vi "Enable Out CHs.vi"(8 "Error In":errorcluster, 9 "Output CH CTL":T1, 10 "OK Button":bool, 11 "UI Refs in":T2) -> (0 "Error Out":errorcluster, 5 "UI Refs out":T2)   [LabVIEW 2017, in "Waveform-Processing-Custom-Device System Explorer.lvlib"]
uses:
  Waveform-Processing-Custom-Device System Explorer.lvlib
  Types/UI Refs Ctl.ctl
  Shared/Types/OutCHEnum.ctl
  Shared/Waveform-Processing-Custom-Device Shared.lvlib
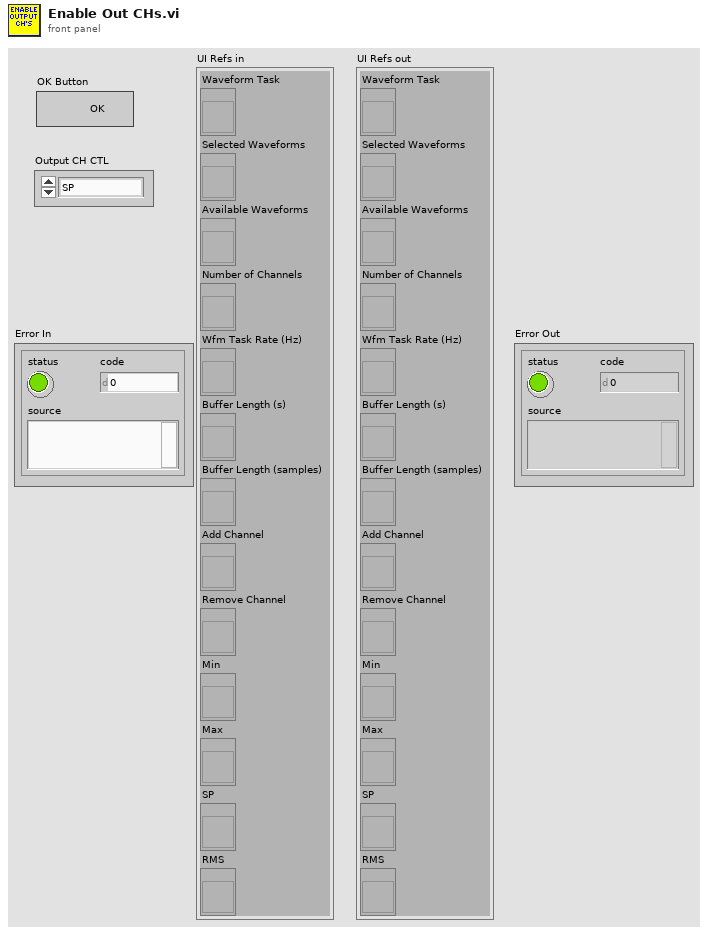
[diagram p1: front panel]
types:
  T1 = typedef "Waveform-Processing-Custom-Device Shared.lvlib/OutCHEnum.ctl" = enum16{"SP", "MIN", "MAX", "RMS"}
  T2 = typedef "Waveform-Processing-Custom-Device Shared.lvlib/UI Refs Ctl.ctl" = cluster{"Waveform Task":refnum<vi>, "Selected Waveforms":refnum<vi>, "Available Waveforms":refnum<vi>, "Number of Channels":refnum<vi>, "Wfm Task Rate (Hz)":refnum<vi>, "Buffer Length (s)":refnum<vi>, "Buffer Length (samples)":refnum<vi>, "Add Channel":refnum<vi>, "Remove Channel":refnum<vi>, "Min":refnum<vi>, "Max":refnum<vi>, "SP":refnum<vi>, "RMS":refnum<vi>}
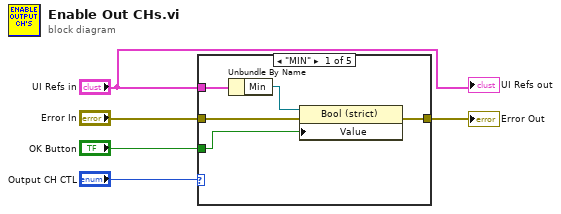
[diagram p0: block diagram]
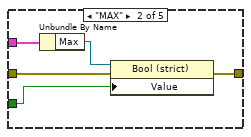
[diagram p2: hidden frame]
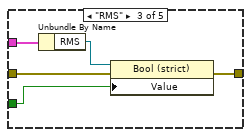
[diagram p3: hidden frame]
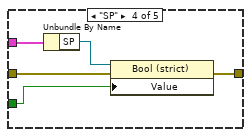
[diagram p4: hidden frame]
diagram:
  n1 = case shown="\"MIN\"" "Output CH CTL" {
    tunnel: "UI Refs in" -> [w10 w15 w20 w25 _]
    tunnel: "Error In" -> [w8 w13 w18 w23 w26]
    tunnel: [w7 w12 w17 w22 w26] -> w3
    tunnel: "OK Button" -> [w6 w11 w16 w21 _]
    frame "MIN" {
      n2 = Unbundle By Name(w10) -> ("Min"=w9:refnum<vi>)
      n3 = property class="Bool (strict)"(reference=w9, error in=w8, "Value"=w6) -> (error out=w7:errorcluster)  [unwired: 1 out]
    }
    frame "MAX" {
      n4 = Unbundle By Name(w15) -> ("Max"=w14:refnum<vi>)
      n5 = property class="Bool (strict)"(reference=w14, error in=w13, "Value"=w11) -> (error out=w12:errorcluster)  [unwired: 1 out]
    }
    frame "RMS" {
      n6 = Unbundle By Name(w20) -> ("RMS"=w19:refnum<vi>)
      n7 = property class="Bool (strict)"(reference=w19, error in=w18, "Value"=w16) -> (error out=w17:errorcluster)  [unwired: 1 out]
    }
    frame "SP" {
      n8 = Unbundle By Name(w25) -> ("SP"=w24:refnum<vi>)
      n9 = property class="Bool (strict)"(reference=w24, error in=w23, "Value"=w21) -> (error out=w22:errorcluster)  [unwired: 1 out]
    }
    frame Default {
    }
  }
  "Error Out" <- w3
  "UI Refs out" <- "UI Refs in"
